vi "PC_Main_SequenceEditor_TempVariable_Initialize.vi"() -> (1 "TempVariable":T2)   [LabVIEW 2010]
uses:
  Ctls/PC_Main_SequenceEditor_TempVariable.ctl
  Ctls/StepData.ctl
panel:
  in  "Sequence":T1[](array[typedef])
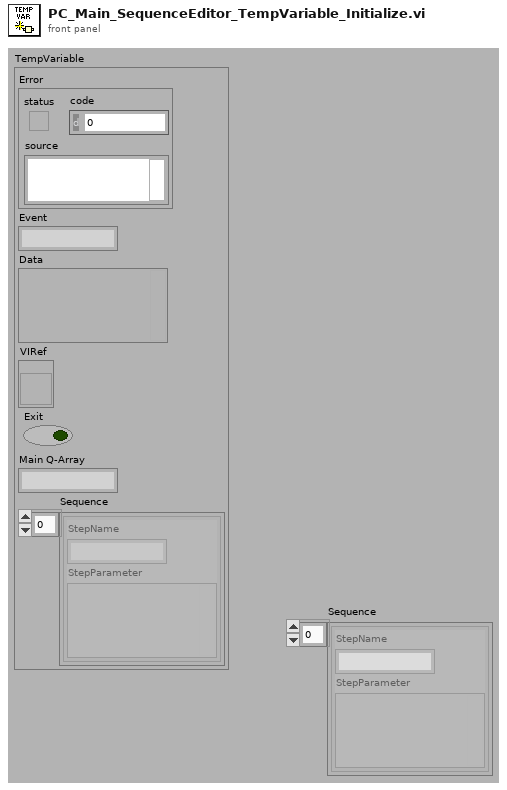
[diagram p1: front panel]
types:
  T1 = typedef "StepData.ctl" = cluster{"StepName":string, "StepParameter":variant}
  T2 = typedef "PC_Main_SequenceEditor_TempVariable.ctl" = cluster{"Error":errorcluster, "Event":string, "Data":variant, "VIRef":refnum<vi>, "Exit":bool, "Main Q-Array":string, "Sequence":T1[]}
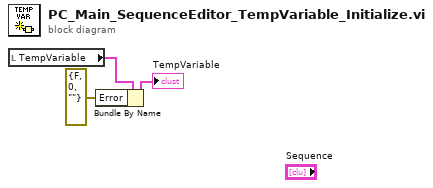
[diagram p0: block diagram]
diagram:
  n1 = local read "TempVariable"() -> (w3:T2)
  n2 = Bundle By Name(cluster=w3, "Error"=errorcluster {"status"=FALSE, "code"=0, "source"=""}) -> (→"TempVariable":T2)
